vi "Send Command.vi"(8 "error in (no error)":errorcluster, 9 "Input Value":string, 10 "Commands":T1, 11 "ESM303 in":refnum<class "ESM303.lvclass">) -> (0 "error out":errorcluster, 3 "ESM303 out":refnum<class "ESM303.lvclass">)   [LabVIEW 2018, in "ESM303.lvlib" / "ESM303.lvclass"]
uses:
  ESM303.lvclass
  builds/Force Test Stand.lvlibp/Custom Controls/Commands.ctl
  builds/Force Test Stand.lvlibp/Force Test Stand.lvclass
  C:/Users/Ron.Dexter.LUMINARTECH/Desktop/builds/Force Test Stand.lvlibp/Force Test Stand.lvclass
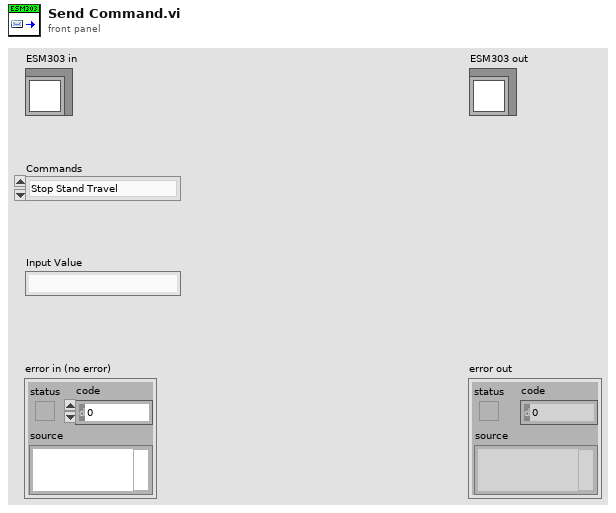
[diagram p1: front panel]
types:
  T1 = typedef "Force Test Stand.lvlibp/Force Test Stand.lvclass/Commands.ctl" = enum16{"Stop Stand Travel", "Start Travel Down (Left)", "Start Travel Up (Right)", "Get Travel Upper Limit", "Get Travel Lower Limit", "Set Travel Upper Limit", "Set Travel Lower Limit", "Get Travel Value", "Set Travel Units (mm)", "Set Travel Units (in)", "Reset Travel to Zero", "Get Speed ", "Set Speed", "Set Speed to Min", "Set Speed to Max", "Get Force Value", "Get Force Units", "Set Force Units (lbF)", "Get Stand Status", "Set Cycle Mode", "Set Limit Mode", "Set Manual Mode", "Set No. Cycles", "Get Travel/Force Values", "Get Completed Cycles", "Get Cycles Setpoint", "Reset Cycles Counter", "Zero Force Gauge", "Set Force Upper Limit", "Set Force Lower Limit", "Get Travel Units", "Get Speed Units", "Default", "Set Force Units (N)", "Set Force Units (kgF)", "Set Force Units (ozF)", "Set Force Units (gF)", "Set Force Real Time Mode", "Set Force Peak Tension Mode", "Set Force Peak Compression Mode", "Set Force High Set-Point", "Set Force Low Set-Point", "Gauge Transmit with Units", "Gauge Transmit w/o Units", "Get Peak Compression Force", "Get Peak Tension Force", "Get Real Time Force", "Disable Force High Limit", "Disable Force Low Limit", "Send Speed Setting to Stand"}
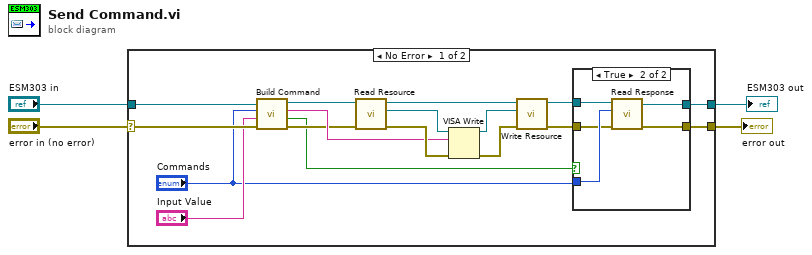
[diagram p0: block diagram]
diagram:
  n1 = case shown="No Error" "error in (no error)" {
    selector: "error in (no error)" -> [w21 w29]
    tunnel: "ESM303 in" -> [w20 w30]
    tunnel: [w12 w30] -> w2
    tunnel: [w13 w29] -> w1
    frame No Error {
      n2 = call "Build Command.vi"("error in"=w21, "Input Value"="Input Value", "Commands"="Commands", "ESM303 in"=w20) -> ("error out"=w15:errorcluster, "Response Expected?"=w5:bool, "Command"=w16:string, "ESM303 out"=w14:refnum<class "ESM303.lvclass">)  [unwired: 4 in]
      n3 = call "Read Resource.vi"("error in (no error)"=w15, "Force Test Stand in"=w14) -> ("error out"=w17:errorcluster, "Resource"=w18:refnum<visa-resource-name>, "Force Test Stand out"=w10:refnum<class "ESM303.lvclass">)  [unwired: 7 in]
      n4 = VISA Write(VISA resource name=w18, write buffer=w16, error in (no error)=w17) -> (VISA resource name out=w6:refnum<visa-resource-name>, error out=w9:errorcluster)  [unwired: 1 out]
      n5 = call "Write Resource.vi"("error in (no error)"=w9, "Resource"=w6, "Force Test Stand in"=w10) -> ("error out"=w7:errorcluster, "Force Test Stand out"=w8:refnum<class "ESM303.lvclass">)  [unwired: 7 in]
      n6 = case shown="True" w5 {
        tunnel: [w22 w28] -> w13
        tunnel: [w23 w27] -> w12
        tunnel: "Commands" -> [_ w26]
        tunnel: w8 -> [w23 w25]
        tunnel: w7 -> [w22 w24]
        frame False {
        }
        frame True {
          n7 = call-dynamic "Read Response.vi"("error in (no error)"=w24, "Commands"=w26, "ESM303 in"=w25) -> ("error out"=w28:errorcluster, "ESM303 out"=w27:refnum<class "ESM303.lvclass">)  [unwired: 7 in]
        }
      }
    }
    frame Error {
    }
  }
  "error out" <- w1
  "ESM303 out" <- w2
